vi "I2C Config Pane.vi"(6 "_SubPanelMessages":refnum<notifier>, 9 "_myEmbeddedToFrameEvent":T6, 10 "_myEmbedded.Exit":refnum<user-event>, 11 "_Property Bundle":cluster{"Name":string, "Value":variant}[](array[cluster])) -> (1 "_Connection Informations":T1, 2 "_Scripter Input":T8)   [LabVIEW 2021]
doc: "Writes data to or reads data from an Inter-Integrated Circuit (I2C) slave device."
uses:
  <vilib>/myRIO/Common/Express VI Framework/xctls/myRIO Channel Name/myRIO Channel Name.xctl
  <vilib>/myRIO/Instrument Drivers/Onboard IO/I2C/typedefs/I2C Transfer Rate.ctl
  <vilib>/myRIO/Common/Express VI Framework/typedefs/Config Pane to Framework Ref.ctl
  <vilib>/myRIO/Common/Express VI Framework/typedefs/Data Validate Ref.ctl
  <vilib>/myRIO/Common/Express VI Framework/typedefs/Scripter Input.ctl
  <vilib>/myRIO/Common/Express VI Framework/typedefs/WireThrough Terminal Names.ctl
  <vilib>/myRIO/Common/Express VI Framework/typedefs/Instrument Driver Method Descriptor Array.ctl
  <vilib>/myRIO/Common/Express VI Framework/typedefs/Instrument Driver Method Descriptor.ctl
  <vilib>/myRIO/Common/Express VI Framework/typedefs/Sub Panel Messages.ctl
  <vilib>/myRIO/Common/Express VI Framework/typedefs/Connection Informations.ctl
  <vilib>/myRIO/Common/Instrument Driver Framework/Utilities/typedefs/Channel Types.ctl
  <vilib>/myRIO/Instrument Drivers/Onboard IO/I2C/typedefs/I2C User Configuration.ctl
  <vilib>/myRIO/Instrument Drivers/Onboard IO/I2C/I2C.lvlib
panel:
  in  "Mode":enum32{"Write", "Read", "Write/Read"}(radio) caption="Mode:"
  in  "Speed:":T2
  out "-Channel Details:":string caption="Connections:"
  in  "Channel:":u16(xcontrol)
  in  "_Default Alias String":string
  in  "_VI Default Name (Edit and make value default)":string="I2C"
  in  "Name:":string caption="Node name:"
  in  "_WireThrough Info (Edit and make value default)":T3={"WireThrough Top In"="I2C Ref In", "WireThrough Bottom In"="error in (no error)", "WireThrough Top Out"="I2C Ref Out", "WireThrough Bottom Out"="error out"}
  in  "_Template Array (Edit and make value default)":T4=[{"Function Name"="Smart Open", "VI Path"=path "<vilib>/myRIO/Instrument Drivers/Onboard IO/I2C/vis", "Script"=TRUE, "Inputs"=[{"name"="Channel Name", "value"=variant, "Config Pane Only"=TRUE, "Build Array"=FALSE, "Bundle Cluster"=FALSE, "Show Term"=FALSE, "alias"=[], "Required Input"=FALSE}], "Outputs"=[], "VI Class"=enum."Open", "Controls Refs[]"=[], "Inline"=FALSE}, {"Function Name"="Open", "VI Path"=path "<vilib>/myRIO/Instrument Drivers/Onboard IO/I2C/vis", "Script"=FALSE, "Inputs"=[{"name"="Channel Name", "value"=variant, "Config Pane Only"=TRUE, "Build Array"=FALSE, "Bundle Cluster"=FALSE, "Show Term"=FALSE, "alias"=[], "Required Input"=FALSE}], "Outputs"=[], "VI Class"=enum."Open", "Controls Refs[]"=[], "Inline"=FALSE}, {"Function Name"="Configure", "VI Path"=path "<vilib>/myRIO/Instrument Drivers/Onboard IO/I2C/vis", "Script"=TRUE, "Inputs"=[{"name"="I2C User Configuration", "value"=variant, "Config Pane Only"=TRUE, "Build Array"=FALSE, "Bundle Cluster"=FALSE, "Show Term"=FALSE, "alias"=[], "Required Input"=FALSE}], "Outputs"=[], "VI Class"=enum."Configure", "Controls Refs[]"=[], "Inline"=FALSE}, {"Function Name"="Write", "VI Path"=path "<vilib>/myRIO/Instrument Drivers/Onboard IO/I2C/vis", "Script"=FALSE, "Inputs"=[{"name"="Slave Address (7-bit)", "value"=variant, "Config Pane Only"=FALSE, "Build Array"=FALSE, "Bundle Cluster"=FALSE, "Show Term"=TRUE, "alias"=[], "Required Input"=TRUE}, {"name"="Bytes to Write", "value"=variant, "Config Pane Only"=FALSE, "Build Array"=FALSE, "Bundle Cluster"=FALSE, "Show Term"=TRUE, "alias"=[], "Required Input"=TRUE}], "Outputs"=[], "VI Class"=enum."Data", "Controls Refs[]"=[], "Inline"=FALSE}, {"Function Name"="Read", "VI Path"=path "<vilib>/myRIO/Instrument Drivers/Onboard IO/I2C/vis", "Script"=FALSE, "Inputs"=[{"name"="Slave Address (7-bit)", "value"=variant, "Config Pane Only"=FALSE, "Build Array"=FALSE, "Bundle Cluster"=FALSE, "Show Term"=TRUE, "alias"=[], "Required Input"=TRUE}, {"name"="Byte Count", "value"=variant, "Config Pane Only"=FALSE, "Build Array"=FALSE, "Bundle Cluster"=FALSE, "Show Term"=TRUE, "alias"=[], "Required Input"=TRUE}], "Outputs"=[{"name"="Bytes Read", "value"=variant, "Show Term"=TRUE, "Index Array"=FALSE, "Unbundle Cluster"=FALSE, "alias"=[]}], "VI Class"=enum."Data", "Controls Refs[]"=[], "Inline"=FALSE}, {"Function Name"="Write Read", "VI Path"=path "<vilib>/myRIO/Instrument Drivers/Onboard IO/I2C/vis", "Script"=FALSE, "Inputs"=[{"name"="Slave Address (7-bit)", "value"=variant, "Config Pane Only"=FALSE, "Build Array"=FALSE, "Bundle Cluster"=FALSE, "Show Term"=TRUE, "alias"=[], "Required Input"=TRUE}, {"name"="Bytes to Write", "value"=variant, "Config Pane Only"=FALSE, "Build Array"=FALSE, "Bundle Cluster"=FALSE, "Show Term"=TRUE, "alias"=[], "Required Input"=TRUE}, {"name"="Byte Count", "value"=variant, "Config Pane Only"=FALSE, "Build Array"=FALSE, "Bundle Cluster"=FALSE, "Show Term"=TRUE, "alias"=[], "Required Input"=TRUE}], "Outputs"=[{"name"="Bytes Read", "value"=variant, "Show Term"=TRUE, "Index Array"=FALSE, "Unbundle Cluster"=FALSE, "alias"=[]}], "VI Class"=enum."Data", "Controls Refs[]"=[], "Inline"=FALSE}, {"Function Name"="Close", "VI Path"=path "<vilib>/myRIO/Instrument Drivers/Onboard IO/I2C/vis", "Script"=FALSE, "Inputs"=[], "Outputs"=[], "VI Class"=enum."Close", "Controls Refs[]"=[], "Inline"=FALSE}]
  in  "_Test Close":bool
  # "User Visible Area"
  # "NOTE: Tab Order has been set\nfor this Front Panel.\n\nSee Edit>>Set Tabbing Order...\n\nAll controls that are not visible at \nruntime are excluded from Tabbing order\n\nTo exlude a control from context\nhelp prefix its label text with a '-'"
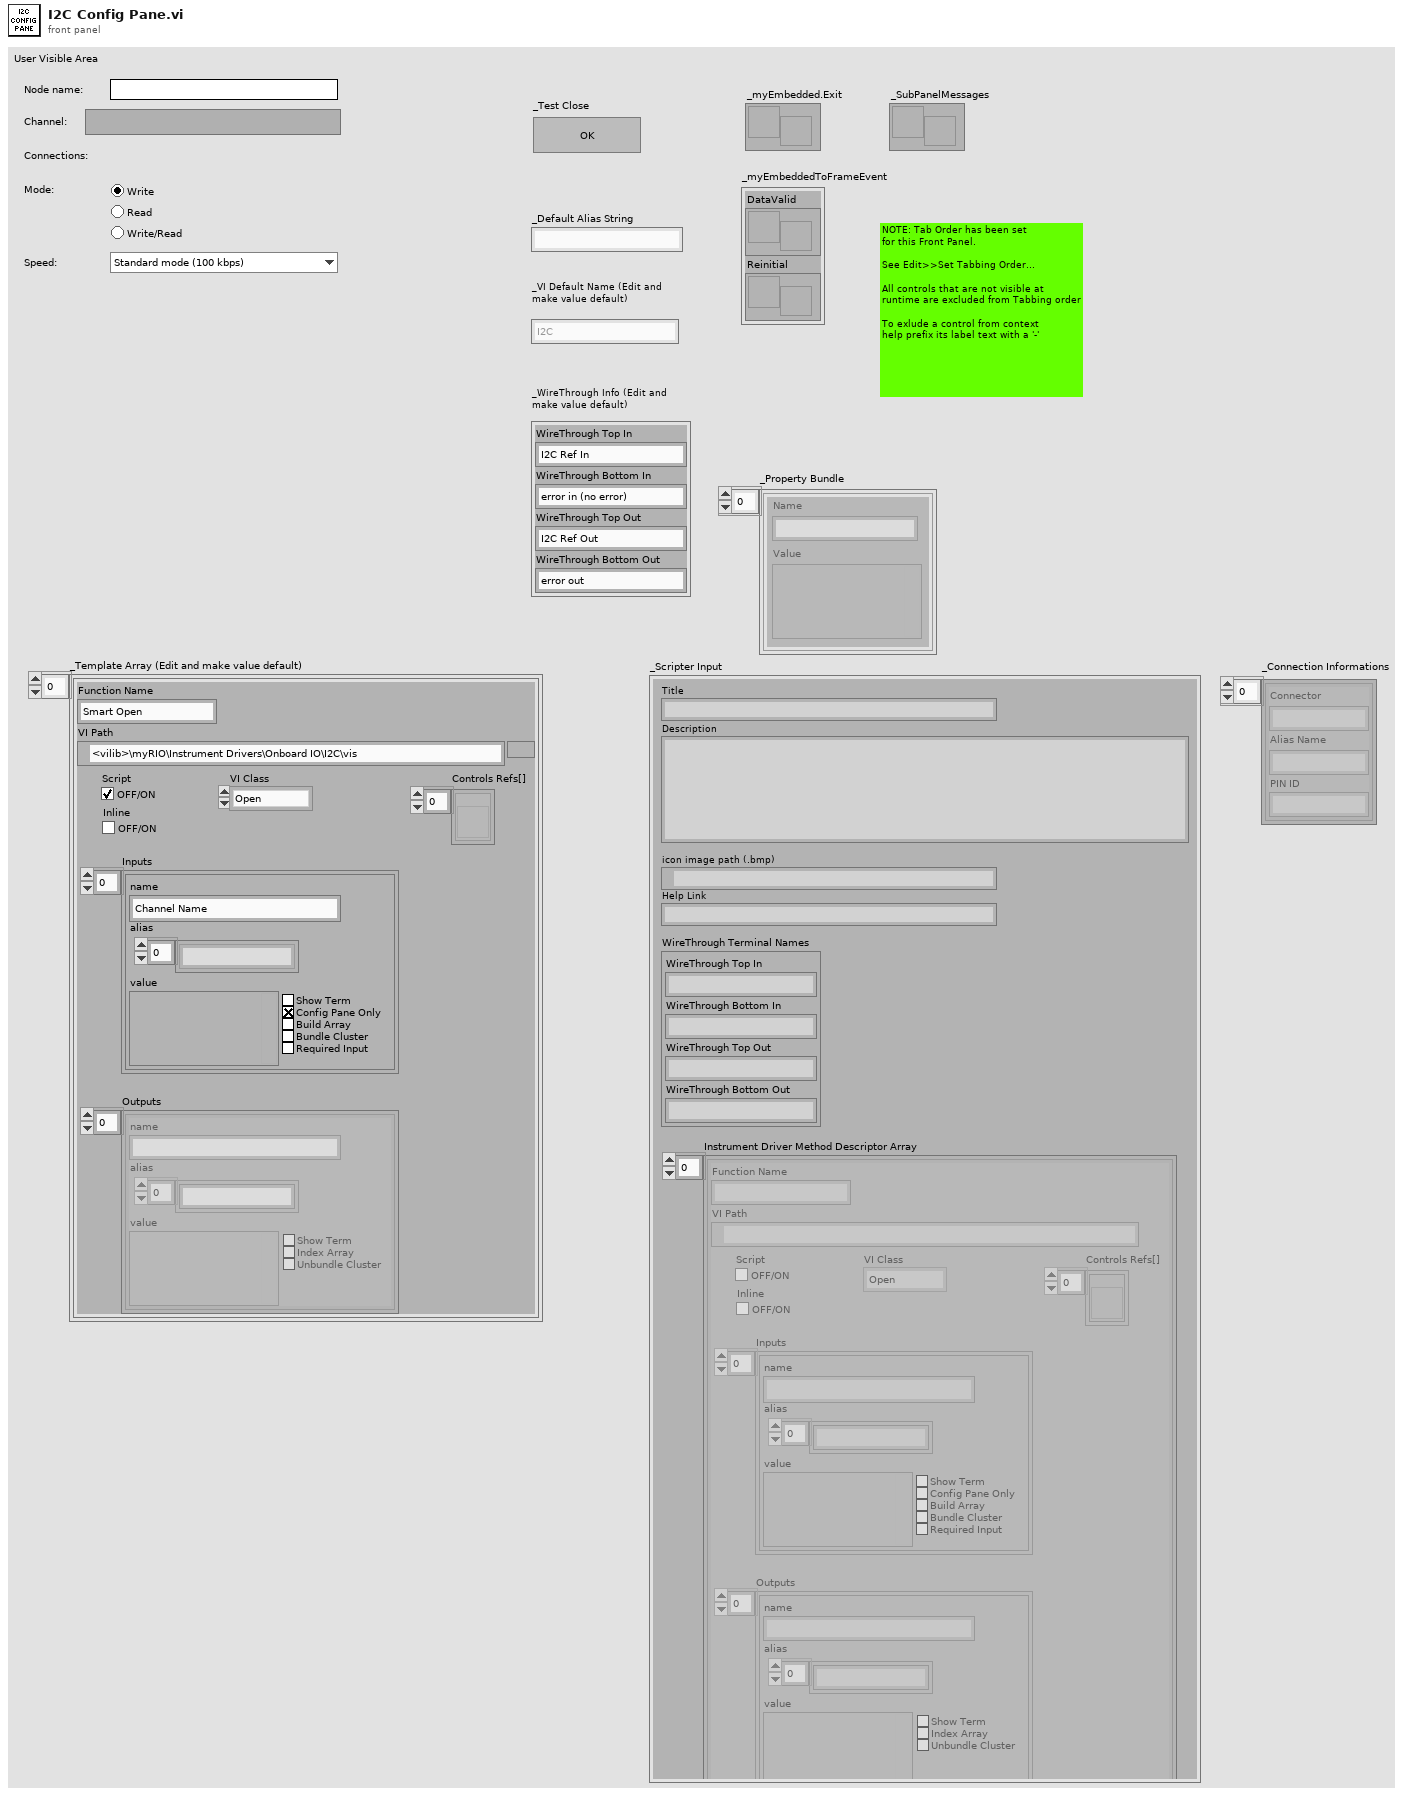
[diagram p1: front panel]
types:
  T1 = typedef "Connection Informations.ctl" = cluster{"Connector":string, "Alias Name":string, "PIN ID":string}[]
  T2 = typedef "I2C.lvlib/I2C Transfer Rate.ctl" = enum16{"Standard mode (100 kbps)", "Fast mode (400 kbps)"}
  T3 = typedef "WireThrough Terminal Names.ctl" = cluster{"WireThrough Top In":string, "WireThrough Bottom In":string, "WireThrough Top Out":string, "WireThrough Bottom Out":string}
  T4 = typedef "Instrument Driver Method Descriptor Array.ctl" = T5[]
  T5 = typedef "Instrument Driver Method Descriptor.ctl" = cluster{"Function Name":string, "VI Path":path, "Script":bool, "Inputs":cluster{"name":string, "value":variant, "Config Pane Only":bool, "Build Array":bool, "Bundle Cluster":bool, "Show Term":bool, "alias":string[], "Required Input":bool}[], "Outputs":cluster{"name":string, "value":variant, "Show Term":bool, "Index Array":bool, "Unbundle Cluster":bool, "alias":string[]}[], "VI Class":enum16{"Open", "Configure", "Data", "Manage", "Close"}, "Controls Refs[]":refnum<vi>[], "Inline":bool}
  T6 = typedef "Config Pane to Framework Ref.ctl" = cluster{"DataValid":T7, "Reinitial":refnum<user-event>}
  T7 = typedef "Data Validate Ref.ctl" = refnum<user-event>
  T8 = typedef "Scripter Input.ctl" = cluster{"Title":string, "Description":string, "icon image path (.bmp)":path, "Help Link":string, "WireThrough Terminal Names":T3, "Instrument Driver Method Descriptor Array":T4}
  T9 = typedef "Channel Types.ctl" = enum32{"Unknown", "AI", "AO", "DIO - DI", "DIO", "DIO - DO", "I2C", "PWM", "Encoder", "SPI", "UART", "Accelerometer", "DIO - LED", "DIO - Button", "AI (N Samples)", "AudioIn (N Samples)", "AO (N Samples)", "AudioOut (N Samples)", "DI (N Samples)", "DO (N Samples)", "AI IRQ", "DI IRQ", "Timer IRQ", "RSL", "Relay", "CAN", "AI (Continuous)", "AO (Continuous)"}
  T10 = typedef "Channel Info.ctl" = cluster{"Channel Name":string, "Alias":string, "Used?":bool, "Not Support?":bool, "Property Bundle":cluster{"Name":string, "Value":variant}[]}
  T11 = typedef "Sub Panel Messages.ctl" = enum16{"Initialized"}
  T12 = cluster{"Connector":string, "Alias Name":string, "PIN ID":string}
  T13 = typedef "I2C.lvlib/I2C User Configuration.ctl" = cluster{"I2C Transfer Rate":T2}
  T14 = cluster{"name":string, "value":variant, "Config Pane Only":bool, "Build Array":bool, "Bundle Cluster":bool, "Show Term":bool, "alias":string[], "Required Input":bool}[]
  T15 = cluster{"name":string, "value":variant, "Config Pane Only":bool, "Build Array":bool, "Bundle Cluster":bool, "Show Term":bool, "alias":string[], "Required Input":bool}
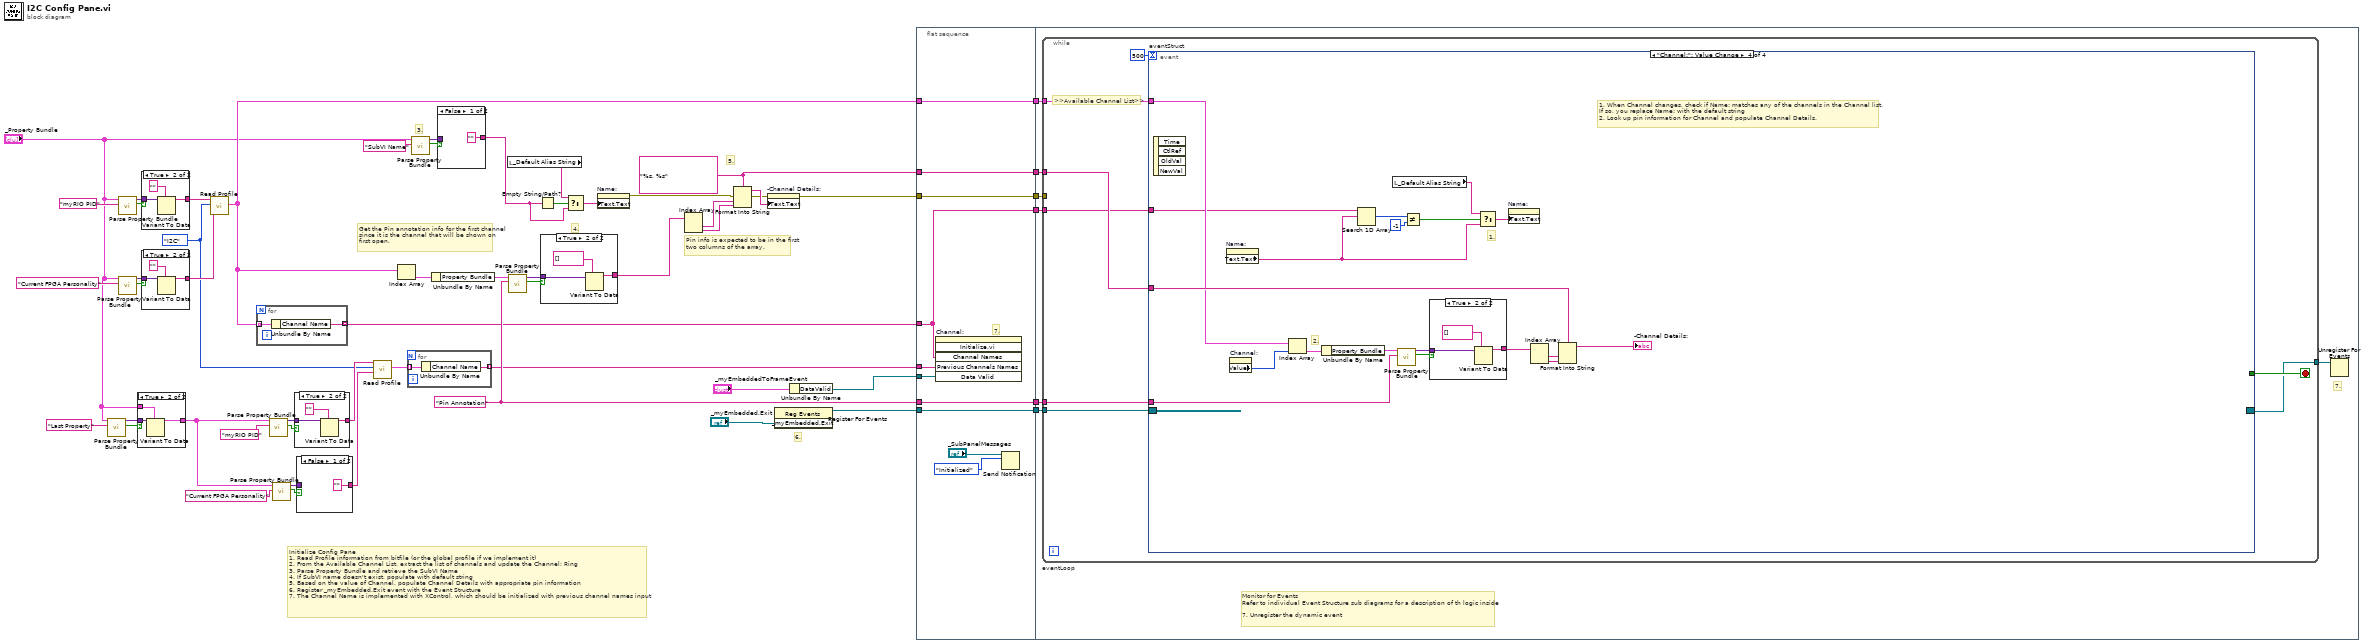
[diagram p0: block diagram]
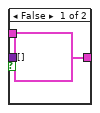
[diagram p2: hidden frame]
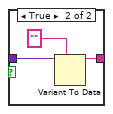
[diagram p3: hidden frame]
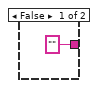
[diagram p4: hidden frame]
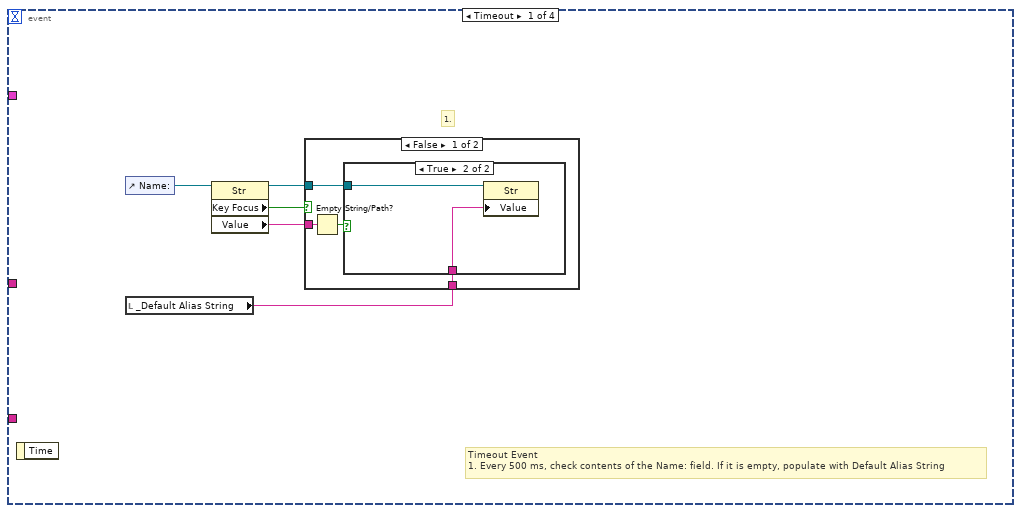
[diagram p5: hidden frame]
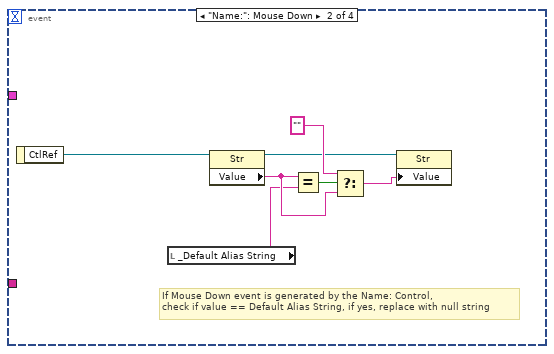
[diagram p8: hidden frame]
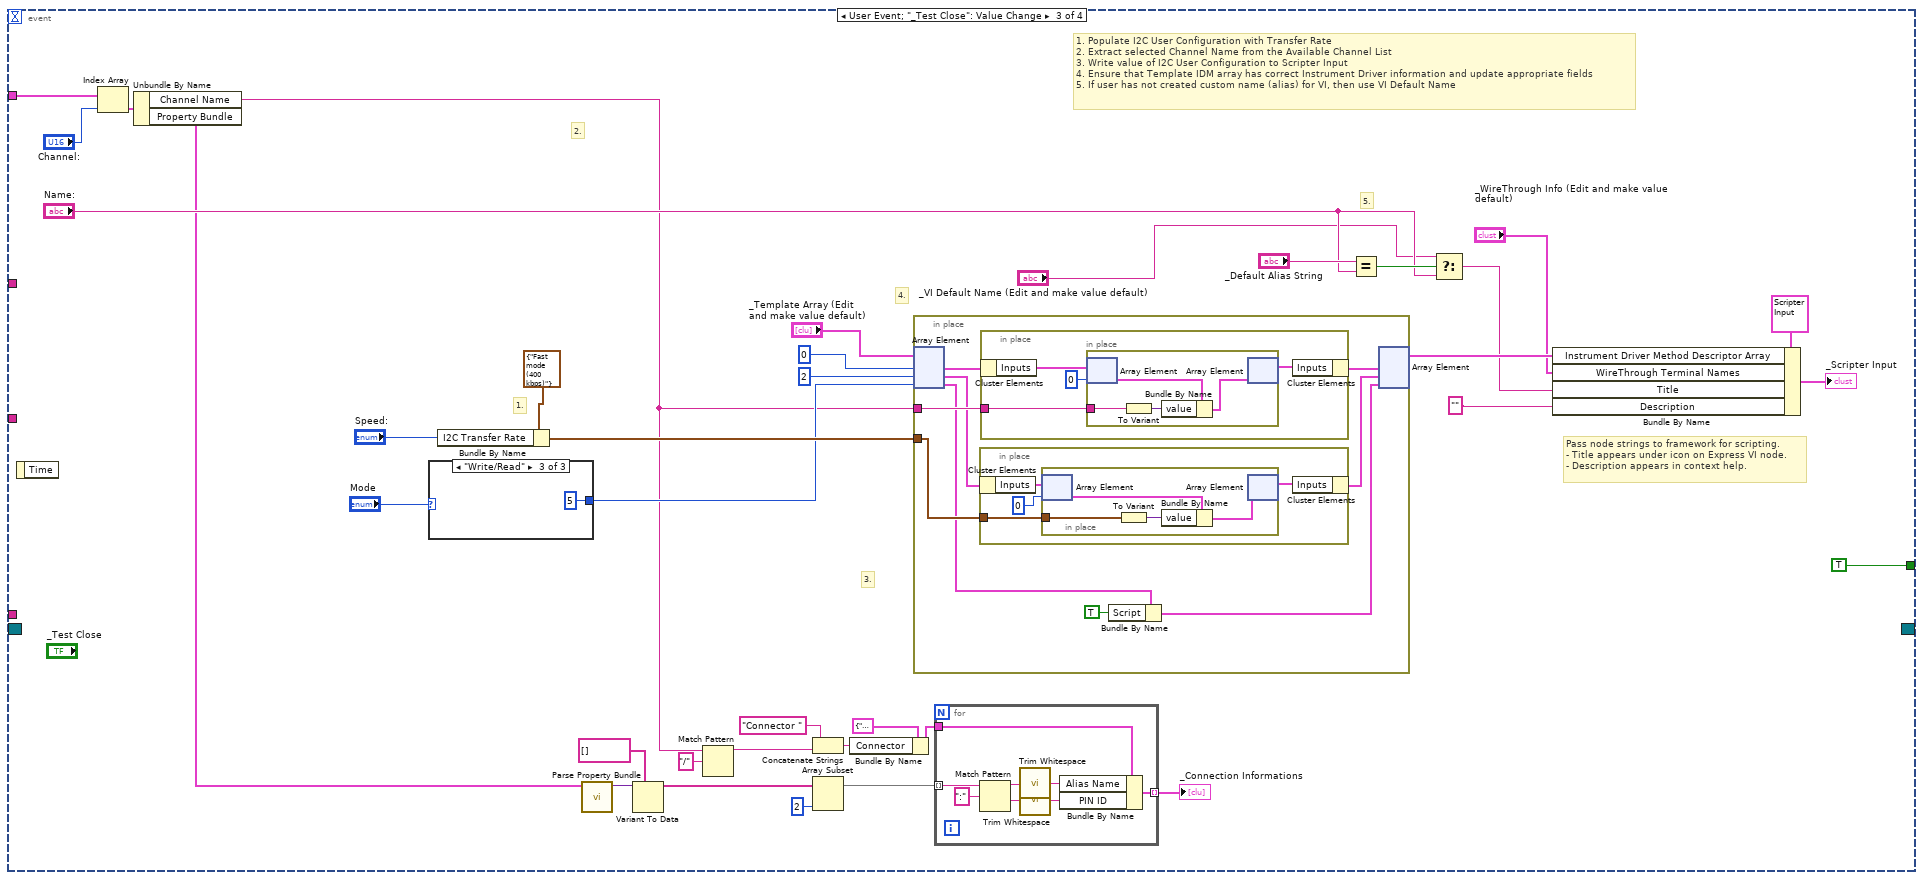
[diagram p9: hidden frame]
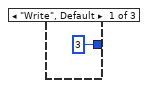
[diagram p10: hidden frame]
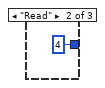
[diagram p11: hidden frame]
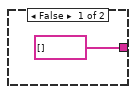
[diagram p12: hidden frame]
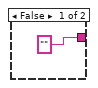
[diagram p13: hidden frame]
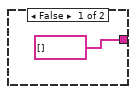
[diagram p14: hidden frame]
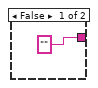
[diagram p15: hidden frame]
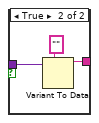
[diagram p16: hidden frame]
diagram:
  w29 = "Pin Annotation" ("Name")
  w4 = Channel_Types."I2C" ("Channel to Read")
  w40 = "%s, %s"
  # "Pin info is expected to be in the first two columns of the array."
  # "Get the Pin annotation info for the first channel  since it is the channel that will be shown on first open."
  # "5."
  # "4."
  # "6."
  # "3."
  # "Initialize Config Pane\n1. Read Profile information from bitfile (or the global profile if we implement it)\n2. From the Available Channel List, extract the list of channels and update the Channel: Ring\n3. Parse Property Bundle and retrieve the SubVI Name\n4. If SubVI name doesn't exist, populate with default string\n5. Based on the value of Channel, populate Channel Details with appropriate pin information\n6. Register _myEmbedded.Exit event with the Event Structure\n7. The Channel Name is implemented with XControl, which should be initialized with previous channel names input"
  n1 = call <vilib>:"Parse Property Bundle.vi"("Name"="Last Property", "Property Bundle"="_Property Bundle") -> ("Found?"=w8:bool, "Value"=w9:variant)  [unwired: 8 in]
  n2 = call <vilib>:"Parse Property Bundle.vi"("Name"="myRIO PID", "Property Bundle"="_Property Bundle") -> ("Found?"=w36:bool, "Value"=w38:variant)  [unwired: 8 in]
  n3 = call <vilib>:"Parse Property Bundle.vi"("Name"="Current FPGA Personality", "Property Bundle"="_Property Bundle") -> ("Found?"=w28:bool, "Value"=w27:variant)  [unwired: 8 in]
  n4 = case shown="True" w8 {
    tunnel: w9 -> [_ w60]
    tunnel: [cluster{"Name":string, "Value":variant}[] [] ("_Property Bundle") w59] -> w7
    tunnel: "_Property Bundle" -> [_ w58]
    frame False {
    }
    frame True {
      n5 = Variant To Data(type=w58, Variant=w60) -> (data=w59:cluster{"Name":string, "Value":variant}[])  [unwired: 1 in, 1 out]
    }
  }
  n6 = case shown="True" w36 {
    tunnel: w38 -> [_ w64]
    tunnel: ["" ("type") w62] -> w37
    frame False {
    }
    frame True {
      n7 = Variant To Data(type="", Variant=w64) -> (data=w62:string)  [unwired: 1 in, 1 out]
    }
  }
  n8 = case shown="True" w28 {
    tunnel: w27 -> [_ w68]
    tunnel: ["" ("type") w66] -> w25
    frame False {
    }
    frame True {
      n9 = Variant To Data(type="", Variant=w68) -> (data=w66:string)  [unwired: 1 in, 1 out]
    }
  }
  n10 = call <vilib>:"Read Profile.vi"("FPGA Name"=w25, "Channel to Read"=w4, "myRIO PID"=w37) -> ("Channel List Out"=w31:T10[])  [unwired: 7 in, 1 out]
  n11 = for {
    tunnel: [w70] -> w2 mode=indexing
    tunnel: w31 -> [w69] mode=indexing
    n12 = Unbundle By Name(w69) -> ("Channel Name"=w70:string)
  }
  n13 = call <vilib>:"Parse Property Bundle.vi"("Name"="myRIO PID", "Property Bundle"=w7) -> ("Found?"=w17:bool, "Value"=w16:variant)  [unwired: 8 in]
  n14 = call <vilib>:"Parse Property Bundle.vi"("Name"="Current FPGA Personality", "Property Bundle"=w7) -> ("Found?"=w12:bool, "Value"=w13:variant)  [unwired: 8 in]
  n15 = case shown="True" w17 {
    tunnel: w16 -> [_ w74]
    tunnel: ["" ("Name") w72] -> w18
    frame False {
    }
    frame True {
      n16 = Variant To Data(type="" ("Name"), Variant=w74) -> (data=w72:string)  [unwired: 1 in, 1 out]
    }
  }
  n17 = case shown="False" w12 {
    tunnel: w13 -> [_ w78]
    tunnel: ["" ("Name") w76] -> w11
    frame False {
    }
    frame True {
      n18 = Variant To Data(type="" ("Name"), Variant=w78) -> (data=w76:string)  [unwired: 1 in, 1 out]
    }
  }
  n19 = call <vilib>:"Read Profile.vi"("FPGA Name"=w11, "Channel to Read"=w4, "myRIO PID"=w18) -> ("Channel List Out"=w6:T10[])  [unwired: 7 in, 1 out]
  n20 = Index Array(array=w31) -> (element=w34:T10)  [unwired: 1 in]
  n21 = for {
    tunnel: [w80] -> w3 mode=indexing
    tunnel: w6 -> [w79] mode=indexing
    n22 = Unbundle By Name(w79) -> ("Channel Name"=w80:string)
  }
  n23 = call <vilib>:"Parse Property Bundle.vi"("Name"="SubVI Name", "Property Bundle"="_Property Bundle") -> ("Found?"=w49:bool, "Value"=w48:variant)  [unwired: 8 in]
  n24 = Unbundle By Name(w34) -> ("Property Bundle"=w35:cluster{"Name":string, "Value":variant}[])
  n25 = case shown="False" w49 {
    tunnel: w48 -> [_ w84]
    tunnel: ["" ("Name") w82] -> w47
    frame False {
    }
    frame True {
      n26 = Variant To Data(type="" ("Name"), Variant=w84) -> (data=w82:string)  [unwired: 1 in, 1 out]
    }
  }
  n27 = local read "_Default Alias String"() -> (w51:string)
  n28 = call <vilib>:"Parse Property Bundle.vi"("Name"=w29, "Property Bundle"=w35) -> ("Found?"=w33:bool, "Value"=w32:variant)  [unwired: 8 in]
  n29 = Empty String/Path?(string/path=w47) -> (empty?=w53:bool)
  n30 = case shown="True" w33 {
    tunnel: w32 -> [_ w88]
    tunnel: [string[] [] w87] -> w30
    frame False {
    }
    frame True {
      n31 = Variant To Data(type=string[] [], Variant=w88) -> (data=w87:string[])  [unwired: 1 in, 1 out]
    }
  }
  n32 = Select(t=w51, s=w53, f=w47) -> (s? t:f=w52:string)
  n33 = property on="Name:" class="Str"("Text.Text"=w52) -> (error out=w46:errorcluster)  [unwired: 2 in, 1 out]
  n34 = Index Array(array=w30) -> (element #1=w42:string, element #2=w41:string)  [unwired: 2 in]
  n35 = Format Into String(format string=w40, error in=w46, w42, w41) -> (resulting string=w45:string, error out=w44:errorcluster)  [unwired: 1 in]
  n36 = property on="-Channel Details:" class="Str"(error in=w44, "Text.Text"=w45) -> (error out=w43:errorcluster)  [unwired: 1 in, 1 out]
  n37 = register-events("_myEmbedded.Exit") -> (reference out=w56:refnum<event-registration>)  [unwired: 2 in, 1 out]
  n38 = Unbundle By Name("_myEmbeddedToFrameEvent") -> ("DataValid"=w24:T7)
  n39 = flat-sequence {
    tunnel: w24 -> [w91]
    tunnel: w29 -> [w94]
    tunnel: w31 -> [w95]
    tunnel: w40 -> [w96]
    tunnel: w43 -> [w97]
    tunnel: w56 -> [w98]
    tunnel: [w98] -> w23
    tunnel: [w97] -> w22
    tunnel: [w96] -> w21
    tunnel: [w95] -> w20
    tunnel: [w94] -> w19
    tunnel: w3 -> [w90]
    tunnel: w2 -> [w89]
    tunnel: [w89] -> w1
    tunnel: w23 -> [w105]
    tunnel: w22 -> [w103]
    tunnel: w21 -> [w102]
    tunnel: w20 -> [w101]
    tunnel: w19 -> [w100]
    tunnel: w1 -> [w99]
    frame #0 {
      # "7."
      n40 = invoke on="Channel:" class="myRIO Channel Name (strict)" method="Initialize.vi"("Channel Names"=w89, "Previous Channels Names"=w90, "Data Valid"=w91) -> ()  [unwired: 3 in, 6 out]
      n41 = Send Notification(notification=Sub_Panel_Messages."Initialized", notifier="_SubPanelMessages") -> ()  [unwired: 1 in, 2 out]
    }
    frame #1 {
      # "7."
      # "Monitor for Events\nRefer to individual Event Structure sub diagrams for a description of th logic inside\n\n7. Unregister the dynamic event"
      n42 = while "eventLoop" {
        tunnel: w105 -> [w112]
        tunnel: [w111] -> w104
        tunnel: w101 -> [w109]
        tunnel: w103 -> [_]
        tunnel: w102 -> [w108]
        tunnel: w100 -> [w107]
        tunnel: w99 -> [w106]
        stop <- w113 stop-if-true
        # ">>Available Channel List>>"
        n43 = event "eventStruct" shown="[3] \"Channel:\": Value Change" {
          selector: w112 -> [_ _ _ _]
          dyn-events: [_ _ _ _] -> w111
          timeout: 500 -> [_ _ _ _]
          tunnel: [_ _ TRUE ("_Test Close") _] -> w113
          tunnel: w109 -> [_ _ w166 w209]
          tunnel: w108 -> [_ _ _ w215]
          tunnel: w107 -> [_ _ _ w210]
          tunnel: w106 -> [_ _ _ w204]
          event Timeout {
            # "Timeout Event\n1. Every 500 ms, check contents of the Name: field. If it is empty, populate with Default Alias String"
            # "1."
            n44 = event-data() -> ()  [unwired: 1 in, 1 out]
            n45 = control-ref of="Name:"() -> (w116:refnum<vi>)
            n46 = local read "_Default Alias String"() -> (w114:string)
            n47 = property on="Property Node" class="Str"(reference=w116) -> (reference out=w115:refnum<vi>, "Key Focus"=w117:bool, "Value"=w118:string)  [unwired: 1 in, 1 out]
            n48 = case shown="False" w117 {
              tunnel: w118 -> [w122 _]
              tunnel: w115 -> [w120 _]
              tunnel: w114 -> [w119 _]
              frame False {
                n49 = Empty String/Path?(string/path=w122) -> (empty?=w121:bool)
                n50 = case shown="True" w121 {
                  tunnel: w120 -> [_ w124]
                  tunnel: w119 -> [_ w123]
                  frame False {
                  }
                  frame True {
                    n51 = property on="Property Node" class="Str"(reference=w124, "Value"=w123) -> ()  [unwired: 1 in, 2 out]
                  }
                }
              }
              frame True {
              }
            }
          }
          event "Name:": Mouse Down {
            # "If Mouse Down event is generated by the Name: Control,\ncheck if value == Default Alias String, if yes, replace with null string"
            n52 = event-data() -> ("CtlRef"=w131:refnum<vi>)  [unwired: 1 in]
            n53 = local read "_Default Alias String"() -> (w125:string)
            n54 = property class="Str"(reference=w131) -> (reference out=w127:refnum<vi>, "Value"=w126:string)  [unwired: 1 in, 1 out]
            n55 = Equal?(x=w126, y=w125) -> (x = y?=w130:bool)
            n56 = Select(t="", s=w130, f=w126) -> (s? t:f=w128:string)
            n57 = property class="Str"(reference=w127, "Value"=w128) -> ()  [unwired: 1 in, 2 out]
          }
          event User Event; "_Test Close": Value Change {
            # "3."
            # "2."
            # "1."
            # "1. Populate I2C User Configuration with Transfer Rate\n2. Extract selected Channel Name from the Available Channel List\n3. Write value of I2C User Configuration to Scripter Input\n4. Ensure that Template IDM array has correct Instrument Driver information and update appropriate fields\n5. If user has not created custom name (alias) for VI, then use VI Default Name"
            # "5."
            # "4."
            # "Pass node strings to framework for scripting.\n- Title appears under icon on Express VI node.\n- Description appears in context help."
            n58 = event-data() -> ()  [unwired: 1 in, 1 out]
            n59 = Index Array(array=w166, index="Channel:") -> (element=w154:T10)
            n60 = Unbundle By Name(w154) -> ("Channel Name"=w137:string, "Property Bundle"=w136:cluster{"Name":string, "Value":variant}[])
            n61 = case shown="\"Write/Read\"" "Mode" {
              tunnel: [3 4 5] -> w148
              frame "Write", Default {
              }
              frame "Read" {
              }
              frame "Write/Read" {
              }
            }
            n62 = Bundle By Name(cluster=T13 {"I2C Transfer Rate"=enum."Fast mode (400 kbps)"} ("I2C User Configuration"), "I2C Transfer Rate"="Speed:") -> (w152:T13)
            n63 = call <vilib>:"Parse Property Bundle.vi"("Property Bundle"=w136) -> ("Value"=w138:variant)  [unwired: 9 in, 1 out]
            n64 = Variant To Data(type=string[] [], Variant=w138) -> (data=w133:string[])  [unwired: 1 in, 1 out]
            n65 = Match Pattern(string=w137, regular expression="/") -> (before substring=w143:string)  [unwired: 1 in, 3 out]
            n66 = Concatenate Strings("Connector " ("string"), w143) -> (w145:string)
            n67 = Array Subset(array=w133, length=2) -> (w134:string[])  [unwired: 1 in]
            n68 = Bundle By Name(cluster=T12 {"Connector"="", "Alias Name"="", "PIN ID"=""} ("Connection Information"), "Connector"=w145) -> (w141:T12)
            n69 = in-place {
              in-place-border: w137 -> [w185]
              in-place-border: w152 -> [w182]
              n70 = in-place-array #1("_Template Array (Edit and make value default)", 0, 2, w148) -> (w187:T5, w184:T5, w181:T5)
              n71 = in-place {
                in-place-border: w182 -> [w188]
                n72 = in-place-cluster #2(w184) -> ("Inputs"=w191:T14)
                n73 = in-place {
                  in-place-border: w188 -> [w193]
                  n74 = in-place-array #3(w191, 0) -> (w195:T15)
                  n75 = To Variant(anything=w193) -> (Variant=w192:variant)
                  n76 = Bundle By Name(cluster=w195, "value"=w192) -> (w194:T15)
                  n77 = in-place-array #3(w194) -> (w190:T14)  [unwired: 1 out]
                }
                n78 = in-place-cluster #2("Inputs"=w190) -> (w183:T5)
              }
              n79 = in-place {
                in-place-border: w185 -> [w198]
                n80 = in-place-cluster #4(w187) -> ("Inputs"=w199:T14)
                n81 = in-place {
                  in-place-border: w198 -> [w200]
                  n82 = in-place-array #5(w199, 0) -> (w203:T15)
                  n83 = To Variant(anything=w200) -> (Variant=w201:variant)
                  n84 = Bundle By Name(cluster=w203, "value"=w201) -> (w202:T15)
                  n85 = in-place-array #5(w202) -> (w197:T14)  [unwired: 1 out]
                }
                n86 = in-place-cluster #4("Inputs"=w197) -> (w186:T5)
              }
              n87 = Bundle By Name(cluster=w181, "Script"=TRUE) -> (w180:T5)
              n88 = in-place-array #1(w186, w183, w180) -> (w164:T4)  [unwired: 3 out]
            }
            n89 = for {
              tunnel: w134 -> [w174] mode=indexing
              tunnel: w141 -> [w175]
              tunnel: [w170] -> w135 mode=indexing
              n90 = Match Pattern(string=w174, regular expression=":") -> (before substring=w172:string, after substring=w171:string)  [unwired: 1 in, 2 out]
              n91 = call <vilib>:"Trim Whitespace.vi"("string"=w172) -> ("trimmed string"=w169:string)  [unwired: 1 in]
              n92 = call <vilib>:"Trim Whitespace.vi"("string"=w171) -> ("trimmed string"=w168:string)  [unwired: 1 in]
              n93 = Bundle By Name(cluster=w175, "Alias Name"=w169, "PIN ID"=w168) -> (w170:T12)
            }
            "_Connection Informations" <- w135
            n94 = Equal?(x="_Default Alias String", y="Name:") -> (x = y?=w156:bool)
            n95 = Select(t="_VI Default Name (Edit and make value default)", s=w156, f="Name:") -> (s? t:f=w155:string)
            n96 = Bundle By Name(cluster=T8 {"Title"="", "Description"="", "icon image path (.bmp)"=path "", "Help Link"="", "WireThrough Terminal Names"={"WireThrough Top In"="", "WireThrough Bottom In"="", "WireThrough Top Out"="", "WireThrough Bottom Out"=""}, "Instrument Driver Method Descriptor Array"=[]} ("Scripter Input"), "Instrument Driver Method Descriptor Array"=w164, "WireThrough Terminal Names"="_WireThrough Info (Edit and make value default)", "Title"=w155, "Description"="" ("Title")) -> (→"_Scripter Input":T8)
          }
          event "Channel:": Value Change {
            # "2."
            # "1."
            # "1. When Channel changes, check if Name: matches any of the channels in the Channel list. \nIf so, you replace Name: with the default string\n2. Look up pin information for Channel and populate Channel Details."
            n97 = event-data() -> ()  [unwired: 1 in, 4 out]
            n98 = property on="Name:" class="Str"() -> ("Text.Text"=w221:string)  [unwired: 2 in, 2 out]
            n99 = property on="Channel:" class="myRIO Channel Name (strict)"() -> ("Value"=w208:u16)  [unwired: 2 in, 2 out]
            n100 = Index Array(array=w209, index=w208) -> (element=w213:T10)
            n101 = Unbundle By Name(w213) -> ("Property Bundle"=w214:cluster{"Name":string, "Value":variant}[])
            n102 = Search 1D Array(1D array=w204, element=w221) -> (index of element=w217:i32)  [unwired: 1 in]
            n103 = local read "_Default Alias String"() -> (w219:string)
            n104 = call <vilib>:"Parse Property Bundle.vi"("Name"=w210, "Property Bundle"=w214) -> ("Found?"=w212:bool, "Value"=w211:variant)  [unwired: 8 in]
            n105 = Not Equal?(x=w217, y=-1) -> (x != y?=w216:bool)
            n106 = case shown="True" w212 {
              tunnel: w211 -> [_ w226]
              tunnel: [string[] [] w225] -> w207
              frame False {
              }
              frame True {
                n107 = Variant To Data(type=string[] [], Variant=w226) -> (data=w225:string[])  [unwired: 1 in, 1 out]
              }
            }
            n108 = Select(t=w219, s=w216, f=w221) -> (s? t:f=w220:string)
            n109 = property on="Name:" class="Str"("Text.Text"=w220) -> ()  [unwired: 2 in, 2 out]
            n110 = Index Array(array=w207) -> (element #1=w206:string, element #2=w205:string)  [unwired: 2 in]
            n111 = Format Into String(format string=w215, w206, w205) -> (resulting string=→"-Channel Details:":string)  [unwired: 2 in, 1 out]
          }
        }
      }
      n112 = Unregister For Events(event registration refnum=w104) -> ()  [unwired: 1 in, 1 out]
    }
  }
